vi "RS232ComPort ReleaseDevice.vi"(8 "error in (no error)":errorcluster, 9 "DeviceIndex":i32=1, 11 "RS232ComPort in":refnum<class "RS232ComPort.lvclass">) -> (0 "error out":errorcluster)   [LabVIEW 2018, in "RS232ComPort.lvclass"]
uses:
  RS232ComPort.lvclass
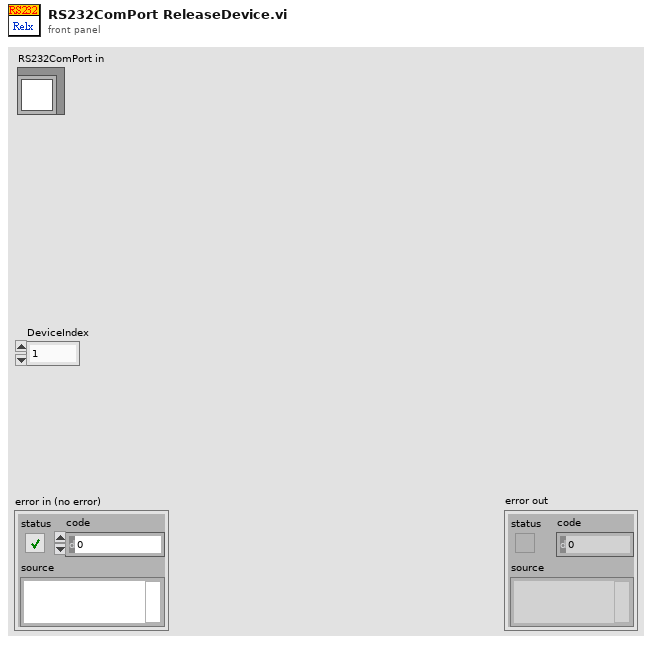
[diagram p1: front panel]
types:
  T1 = typedef "Semaphore RefNum" = refnum<k1>
  T2 = cluster{"Response Str":string, "VISA resource":refnum<visa-resource-name>, "DeviceExist?":bool, "semaphore":T1}
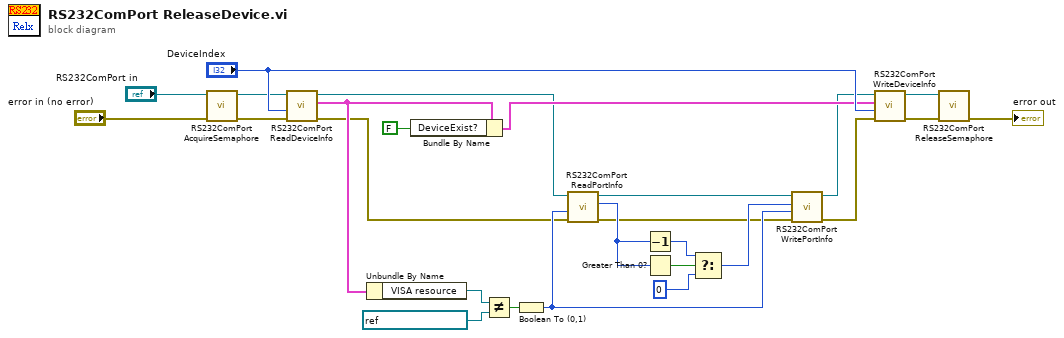
[diagram p0: block diagram]
diagram:
  n1 = call-dynamic "RS232ComPort AcquireSemaphore.vi"("error in (no error)"="error in (no error)", "RS232ComPort in"="RS232ComPort in") -> ("error out"=w7:errorcluster, "RS232ComPort out"=w8:refnum<class "RS232ComPort.lvclass">)  [unwired: 8 in]
  n2 = call-dynamic "RS232ComPort ReadDeviceInfo.vi"("error in (no error)"=w7, "DeviceIndex"="DeviceIndex", "RS232ComPort in"=w8) -> ("error out"=w1:errorcluster, "DeviceInfo"=w16:T2, "RS232ComPort out"=w22:refnum<class "RS232ComPort.lvclass">)  [unwired: 6 in]
  n3 = Unbundle By Name(w16) -> ("VISA resource"=w18:refnum<visa-resource-name>)
  n4 = Bundle By Name(cluster=w16, "DeviceExist?"=FALSE) -> (w25:T2)
  n5 = Not Equal?(x=w18, y=refnum<visa-resource-name> "ASRL1::INSTR" ("VISA resource name")) -> (x != y?=w20:bool)
  n6 = Boolean To (0,1)(Boolean=w20) -> (0, 1=w21:i16)
  n7 = call-dynamic "RS232ComPort ReadPortInfo.vi"("error in (no error)"=w1, "Channel"=w21, "RS232ComPort in"=w22) -> ("error out"=w3:errorcluster, "Status"=w13:i8, "RS232ComPort out"=w23:refnum<class "RS232ComPort.lvclass">)  [unwired: 6 in]
  n8 = Decrement(x=w13) -> (x-1=w15:i8)
  n9 = Greater Than 0?(x=w13) -> (x > 0?=w12:bool)
  n10 = Select(t=w15, s=w12, f=i8 0) -> (s? t:f=w14:i8)
  n11 = call-dynamic "RS232ComPort WritePortInfo.vi"("error in (no error)"=w3, "Channel"=w21, "Status"=w14, "RS232ComPort in"=w23) -> ("error out"=w4:errorcluster, "RS232ComPort out"=w24:refnum<class "RS232ComPort.lvclass">)  [unwired: 6 in]
  n12 = call-dynamic "RS232ComPort WriteDeviceInfo.vi"("error in (no error)"=w4, "DeviceIndex"="DeviceIndex", "DeviceInfo"=w25, "RS232ComPort in"=w24) -> ("error out"=w9:errorcluster, "RS232ComPort out"=w10:refnum<class "RS232ComPort.lvclass">)  [unwired: 6 in]
  n13 = call-dynamic "RS232ComPort ReleaseSemaphore.vi"("error in (no error)"=w9, "RS232ComPort in"=w10) -> ("error out"=→"error out":errorcluster)  [unwired: 8 in, 1 out]
